vi "TKPS252XG Output on-off24.vi"(2 "error in (no error)":errorcluster, 3 "output (t:on)":bool=TRUE, 4 "VISA session":refnum<visa-resource-name>) -> (0 "error out":errorcluster, 1 "dup VISA session":refnum<visa-resource-name>)   [LabVIEW 2024]
doc: "This vi enables/disables the output signal of the power supply."
panel:
  # "on"
  # "off"
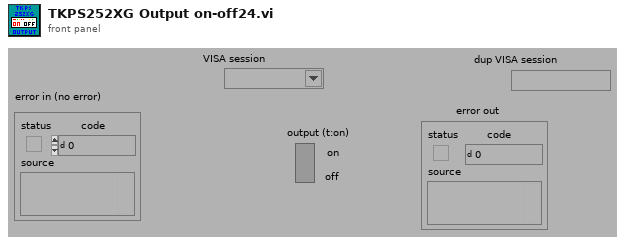
[diagram p1: front panel]
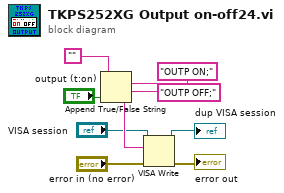
[diagram p0: block diagram]
diagram:
  n1 = Append True/False String(1:"output (t:on)", 2:"OUTP OFF;", 3:"OUTP ON;", 4:"") -> (0:w6:string)
  n2 = VISA Write(VISA resource name="VISA session", write buffer=w6, error in (no error)="error in (no error)") -> (VISA resource name out=→"dup VISA session":refnum<visa-resource-name>, error out=→"error out":errorcluster)  [unwired: 1 out]
